vi "configure.vi"(8 "error in (no error)":errorcluster, 9 "timeStamp":string, 10 "Path":path, 11 "BECHWCBasic in":refnum<class "BECHWCBasic.lvclass">) -> (0 "error out":errorcluster, 3 "BECHWCBasic out":refnum<class "BECHWCBasic.lvclass">)   [LabVIEW 2009, in "Hardware.lvlib" / "HWControllers.lvlib" / "BECHWCBasic.lvclass"]
uses:
  BECHWCBasic.lvclass
  Channels/Digital/DigitalOutput.lvclass
  Channels/VoltOutput/AnalogOutput.lvclass
  HWController.lvclass
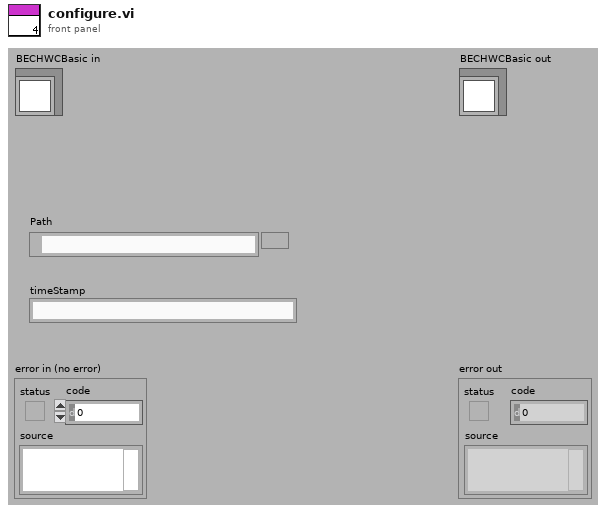
[diagram p1: front panel]
types:
  T1 = enum16{"Ready", "Compiling", "Configured", "Running", "Stopping", "Unresolved Error"}
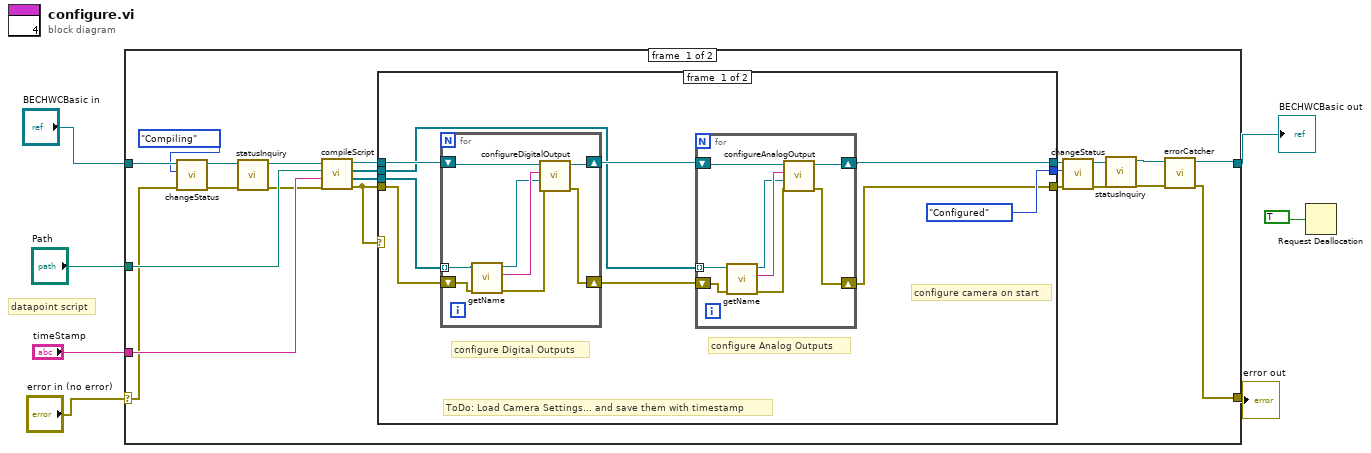
[diagram p0: block diagram]
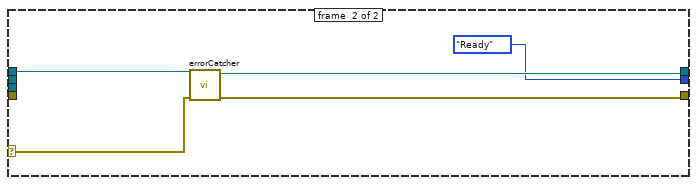
[diagram p2: hidden frame]
diagram:
  # "datapoint script"
  n1 = case shown="No Error" "error in (no error)" {
    selector: "error in (no error)" -> [w14 w60]
    tunnel: "BECHWCBasic in" -> [w18 w61]
    tunnel: [w10 w61] -> w6
    tunnel: [w8 w60] -> w4
    tunnel: "Path" -> [w22 _]
    tunnel: "timeStamp" -> [w21 _]
    frame #0 {
      n2 = call "changeStatus.vi"("error in (no error)"=w14, "status"=T1."Compiling", "HWController in"=w18) -> ("error out"=w20:errorcluster, "HWController out"=w19:refnum<class "BECHWCBasic.lvclass">)  [unwired: 7 in]
      n3 = call-dynamic "statusInquiry.vi"("error in (no error)"=w20, "HWController in"=w19) -> ("error out"=w16:errorcluster, "HWController out"=w17:refnum<class "BECHWCBasic.lvclass">)  [unwired: 8 in]
      n4 = call "compileScript.vi"("error in (no error)"=w16, "timeStamp"=w21, "Path"=w22, "HWController in"=w17) -> ("error out"=w13:errorcluster, "doChannels"=w24:refnum<class "DigitalOutput.lvclass">[], "aoChannels"=w23:refnum<class "AnalogOutput.lvclass">[], "HWController out"=w25:refnum<class "BECHWCBasic.lvclass">)  [unwired: 4 in]
      n5 = case shown="No Error" w13 {
        selector: w13 -> [_ w56]
        tunnel: [w31 w58] -> w29
        tunnel: [w30 w57] -> w28
        tunnel: w25 -> [w37 w59]
        tunnel: w13 -> [w36 _]
        tunnel: w24 -> [w34 _]
        tunnel: w23 -> [w33 _]
        tunnel: [T1."Configured" ("status") T1."Ready" ("status")] -> w12
        frame #0 {
          # "configure camera on start"
          # "ToDo: Load Camera Settings... and save them with timestamp"
          # "configure Analog Outputs"
          # "configure Digital Outputs"
          n6 = for {
            shift-right: [w48] -> w35
            shift-left: w36 -> [w54]
            shift-right: [w52] -> w38
            shift-left: w37 -> [w53]
            tunnel: w34 -> [w47] mode=indexing
            n7 = call-dynamic "getName.vi"("error in (no error)"=w54, "DigitalOutput.lvclass in"=w47) -> ("error out"=w50:errorcluster, "name"=w51:string, "DigitalOutput.lvclass out"=w49:refnum<class "DigitalOutput.lvclass">)  [unwired: 7 in]
            n8 = call "configureDigitalOutput.vi"("error in (no error)"=w50, "DigitalOutput"=w49, "deviceName"=w51, "BECHWCBasic in"=w53) -> ("error out"=w48:errorcluster, "BECHWCBasic out"=w52:refnum<class "BECHWCBasic.lvclass">)  [unwired: 6 in]
          }
          n9 = for {
            tunnel: w33 -> [w39] mode=indexing
            shift-right: [w43] -> w30
            shift-left: w35 -> [w46]
            shift-right: [w44] -> w31
            shift-left: w38 -> [w45]
            n10 = call "getName.vi"("error in (no error)"=w46, "AnalogOutput.lvclass in"=w39) -> ("error out"=w42:errorcluster, "name"=w41:string, "AnalogOutput.lvclass out"=w40:refnum<class "AnalogOutput.lvclass">)  [unwired: 7 in]
            n11 = call "configureAnalogOutput.vi"("error in (no error)"=w42, "AnalogOutput"=w40, "deviceName"=w41, "BECHWCBasic in"=w45) -> ("error out"=w43:errorcluster, "BECHWCBasic out"=w44:refnum<class "BECHWCBasic.lvclass">)  [unwired: 6 in]
          }
        }
        frame #1 {
          n12 = call-dynamic "errorCatcher.vi"("error in (no error)"=w56, "HWController in"=w59) -> ("error out"=w57:errorcluster, "HWController out"=w58:refnum<class "BECHWCBasic.lvclass">)  [unwired: 8 in]
        }
      }
      n13 = call "changeStatus.vi"("error in (no error)"=w28, "status"=w12, "HWController in"=w29) -> ("error out"=w27:errorcluster, "HWController out"=w26:refnum<class "BECHWCBasic.lvclass">)  [unwired: 7 in]
      n14 = call-dynamic "statusInquiry.vi"("error in (no error)"=w27, "HWController in"=w26) -> ("error out"=w9:errorcluster, "HWController out"=w11:refnum<class "BECHWCBasic.lvclass">)  [unwired: 8 in]
      n15 = call-dynamic "errorCatcher.vi"("error in (no error)"=w9, "HWController in"=w11) -> ("error out"=w8:errorcluster, "HWController out"=w10:refnum<class "BECHWCBasic.lvclass">)  [unwired: 8 in]
    }
    frame #1 {
    }
  }
  "error out" <- w4
  "BECHWCBasic out" <- w6
  n16 = Request Deallocation(TRUE) -> ()
